vi "HFRR ADV v08 new software.vi"() -> ()   [LabVIEW 2025] (continued)
                n2706 = local read "String 37"() -> (w3531:string)
                n2707 = local read "String 36"() -> (w3528:string)
                n2708 = local read "String 38"() -> (w3525:string)
                n2709 = local read "String 39"() -> (w3522:string)
                n2710 = Match Pattern(string=w3552, regular expression=".dwm") -> (before substring=w3548:string)  [unwired: 1 in, 3 out]
                "before substring" <- w3548
                n2711 = local read "S 38"() -> (w3543:string)
                n2712 = local read "S 39"() -> (w3536:string)
                n2713 = local read "Temperature before test 2"() -> (w3572:dbl)
                n2714 = local read "Temperature after test 2"() -> (w3577:dbl)
                n2715 = local read "Humidity before test 2"() -> (w3558:dbl)
                n2716 = local read "Humidity after test 2"() -> (w3573:dbl)
                n2717 = local read "MWSD 2"() -> (w3569:dbl)
                n2718 = local read "WS1.4 2"() -> (w3585:dbl)
                n2719 = local read "HCF 2"() -> (w3581:dbl)
                n2720 = local read "AVP 2"() -> (w3570:dbl)
                n2721 = Concatenate Strings("1," ("string"), w3543) -> (w3542:string)
                n2722 = Concatenate Strings("2," ("string"), w3540) -> (w3539:string)
                n2723 = Concatenate Strings("3," ("string"), w3536) -> (w3538:string)
                n2724 = Concatenate Strings("4," ("string"), w3535) -> (w3534:string)
                n2725 = Concatenate Strings("5," ("string"), w3531) -> (w3532:string)
                n2726 = Concatenate Strings("6," ("string"), w3528) -> (w3529:string)
                n2727 = Concatenate Strings("7," ("string"), w3525) -> (w3526:string)
                n2728 = Concatenate Strings("8," ("string"), w3522) -> (w3523:string)
                n2729 = local read "Sample ID"() -> (w3590:string)
                n2730 = case shown="\"xlx\"" "Select File Type" {
                  tunnel: w3548 -> [w3593 w3595 w3597]
                  tunnel: [w3591 w3596 w3598] -> w3547
                  frame "xlx" {
                    n2731 = Concatenate Strings(w3593, ".xls" ("string")) -> (w3591:string)
                  }
                  frame "csv" {
                    n2732 = Concatenate Strings(w3595, ".csv" ("string")) -> (w3596:string)
                  }
                  frame "txt" {
                    n2733 = Concatenate Strings(w3597, ".txt" ("string")) -> (w3598:string)
                  }
                }
                n2734 = local read "Test Date"() -> (w3589:string)
                n2735 = local read "String 45"() -> (w3503:string)
                n2736 = local read "String 31"() -> (w3588:string)
                n2737 = local read "String 32"() -> (w3587:string)
                n2738 = local read "TITTLE"() -> (w3511:string)
                n2739 = Number To Fractional String(number=w3558, width (-)=i16 6, precision (6)=i16 2) -> (F-format string=w3557:string)  [unwired: 1 in]
                n2740 = Number To Fractional String(number=w3572, width (-)=i16 6, precision (6)=i16 2) -> (F-format string=w3578:string)  [unwired: 1 in]
                n2741 = Number To Fractional String(number=w3573, width (-)=i16 6, precision (6)=i16 2) -> (F-format string=w3571:string)  [unwired: 1 in]
                n2742 = Number To Fractional String(number=w3577, width (-)=i16 6, precision (6)=i16 2) -> (F-format string=w3576:string)  [unwired: 1 in]
                n2743 = Number To Fractional String(number=w3569, width (-)=i16 6, precision (6)=i16 2) -> (F-format string=w3567:string)  [unwired: 1 in]
                n2744 = Number To Fractional String(number=w3570, width (-)=i16 6, precision (6)=i16 2) -> (F-format string=w3568:string)  [unwired: 1 in]
                n2745 = Number To Fractional String(number=w3581, width (-)=i16 6, precision (6)=i16 2) -> (F-format string=w3582:string)  [unwired: 1 in]
                n2746 = Number To Fractional String(number=w3585, precision (6)=i16 2) -> (F-format string=w3586:string)  [unwired: 2 in]
                n2747 = local read "s.NO"() -> (w3505:string)
                n2748 = Concatenate Strings("=" ("string"), w3511) -> (w3510:string)
                n2749 = Concatenate Strings("S.No," ("string"), "                                       Parameters" ("string")) -> (w3516:string)
                n2750 = Concatenate Strings(w3583, w3542, w3557, w3583, w3539, w3578, w3583, w3538, w3571, w3583, w3534, w3576, w3583, w3532, w3567, w3583, w3529, w3568, w3583, w3526, w3582, w3583, w3523, w3586) -> (w3545:string)
                n2751 = Concatenate Strings(w3515, "," ("string"), w3503, w3505, w3504, w3587, w3590, w3504, w3588, w3589, w3515) -> (w3513:string)
                n2752 = local read "Tested by"() -> (w3519:string)
                n2753 = local read "String 33"() -> (w3520:string)
                n2754 = Concatenate Strings("," ("string"), "                                                                             " ("string")) -> (w3508:string)
                n2755 = Concatenate Strings(w3510, w3506, w3513, w3506, w3516, w3545, w3506, w3508, w3520, w3519) -> (→"export":string)
                n2756 = String To Path(string=w3547) -> (path=w3554:path)
                n2757 = local read "export"() -> (w3549:string)
                n2758 = call <vilib>:"Write Characters To File.vi"("append to file? (new file:F)"=FALSE, "character string"=w3549, "file path (dialog if empty)"=w3554) -> ()  [unwired: 2 in, 1 out]
              }
            }
          }
          frame Enabled {
          }
        }
        n2759 = case shown="True" "OK Button 17" {
          frame False {
          }
          frame True {
            (unwired) 0  # existing file
            w3807 = "Choose a datalog file to open"  # prompt
            n2760 = local write "OK Button 17"(FALSE ("OK Button 17")) -> ()
            n2761 = local read "String"() -> (w3802:string)
            n2762 = String To Path(string=w3802) -> (path=w3803:path)
            n2763 = File Dialog(6:"*.duf" ("pattern"), 7:w3807, 11:w3803) -> (0:w3794:errorcluster, 3:w3813:path)  [unwired: 4 in, 2 out]
            n2764 = Unbundle(w3794) -> ()  [unwired: 3 out]
            n2765 = Open/Create/Replace File "Open File"(file path (use dialog)=w3813) -> (refnum out=w3805:refnum<file>)  [unwired: 5 in, 2 out]
            n2766 = Strip Path(path=w3813) -> (name=w3811:string)  [unwired: 1 out]
            n2767 = Path To String(path=w3813) -> (string=w3796:string)
            n2768 = while {
              tunnel: w3805 -> [w3817]
              i -> [w3814]
              stop <- w3815 continue-if-true
              (unwired) TRUE ("line mode (F)")
              n2769 = Read from Text File "Read File"(file (use dialog)=w3817) -> (text=w3816:string)  [unwired: 3 in, 3 out]
              n2770 = local write "Numeric 16"(w3814) -> ()
              n2771 = String Length(string=w3816) -> (length=w3819:i32)
              n2772 = Greater?(x=w3819, y=1) -> (0:w3815:bool)
            }
            n2773 = local write "String 29"(w3796) -> ()
            n2774 = Search and Replace String(input string=w3796, search string=".duf", replace string=".dgf" ("replace string (\"\")")) -> (result string=→"String Indicator 4":string)  [unwired: 5 in, 3 out]
            n2775 = Match Pattern(string=w3811, regular expression=".dwm") -> (before substring=w3795:string)  [unwired: 1 in, 3 out]
            "String Indicator" <- w3795
            n2776 = Match Pattern(string=w3796, regular expression=".dwm" ("substring (\"\")")) -> (before substring=w3797:string)  [unwired: 1 in, 3 out]
            "String Indicator 3" <- w3797
            n2777 = local write "TITTLE 2"(w3795) -> ()
            n2778 = String To Path(string=w3797) -> (path=w3804:path)
            "path" <- w3804
            n2779 = call <vilib>:"Read Characters From File.vi"("file path (dialog if empty)"=w3804, "start of read offset (chars.:0)"=60 ("start of read offset (chars.: 0)")) -> ("character string"=→"String Indicator 2":string)  [unwired: 4 in, 3 out]
          }
        }
        n2780 = call <vilib>:"Query Available Printers.vi"() -> ("system configured printers"=w3496:string[])  [unwired: 9 in, 2 out]
        "System Configured Printers 2" <- w3496
        n2781 = local read "OK Button 16"() -> (w3493:bool)
        n2782 = case shown="True" "OK Button 16" {
          frame False {
          }
          frame True {
            n2783 = stacked-sequence {
              frame #0 {
                n2784 = local read "Numeric 16"() -> (w3821:i32)
                n2785 = local write "Numeric 10"(w3821) -> ()
              }
              frame #1 {
                n2786 = local read "S.NO"() -> (→"s.NO":string)
                n2787 = local read "String 29"() -> (w3825:string)
                n2788 = String To Path(string=w3825) -> (path=w3824:path)
                n2789 = Open/Create/Replace File "Open File"(file path (use dialog)=w3824) -> (refnum out=w3826:refnum<file>)  [unwired: 5 in, 2 out]
                n2790 = for {
                  N: 16 -> [_]
                  tunnel: w3826 -> [w3833]
                  i -> [w3829]
                  (unwired) TRUE ("line mode (F)")
                  n2791 = Read from Text File "Read File"(file (use dialog)=w3833) -> (text=w3827:string)  [unwired: 3 in, 3 out]
                  n2792 = Match Pattern(string=w3827, regular expression="(") -> (after substring=w3832:string)  [unwired: 1 in, 3 out]
                  n2793 = Match Pattern(string=w3832, regular expression=")") -> (before substring=w3828:string)  [unwired: 1 in, 3 out]
                  n2794 = case shown="1" w3829 {
                    tunnel: w3828 -> [w3834 w3835 _ _ w3836 w3837 w3838 w3840 w3842 w3844 w3846 w3848 w3850 w3852 _]
                    tunnel: w3827 -> [_ _ _ _ _ _ _ _ _ _ _ _ _ _ _]
                    frame 0 {
                      "TITTLE" <- w3834
                    }
                    frame 1 {
                      "Sample ID" <- w3835
                    }
                    frame 2 {
                    }
                    frame 3 {
                    }
                    frame 4 {
                      "Test Date" <- w3836
                    }
                    frame 5 {
                      "Tested by" <- w3837
                    }
                    frame 6 {
                      n2795 = Fract/Exp String To Number(string=w3838) -> (number=→"Humidity before test 2":dbl)  [unwired: 3 in, 1 out]
                    }
                    frame 7 {
                      n2796 = Fract/Exp String To Number(string=w3840) -> (number=→"Temperature before test 2":dbl)  [unwired: 3 in, 1 out]
                    }
                    frame 8 {
                      n2797 = Fract/Exp String To Number(string=w3842) -> (number=→"Humidity after test 2":dbl)  [unwired: 3 in, 1 out]
                    }
                    frame 9 {
                      n2798 = Fract/Exp String To Number(string=w3844) -> (number=→"Temperature after test 2":dbl)  [unwired: 3 in, 1 out]
                    }
                    frame 10 {
                      n2799 = Fract/Exp String To Number(string=w3846) -> (number=→"MWSD 2":dbl)  [unwired: 3 in, 1 out]
                    }
                    frame 11 {
                      n2800 = Fract/Exp String To Number(string=w3848) -> (number=→"AVP 2":dbl)  [unwired: 3 in, 1 out]
                    }
                    frame 12 {
                      n2801 = Fract/Exp String To Number(string=w3850) -> (number=→"HCF 2":dbl)  [unwired: 3 in, 1 out]
                    }
                    frame 13 {
                      n2802 = Fract/Exp String To Number(string=w3852) -> (number=→"WS1.4 2":dbl)  [unwired: 3 in, 1 out]
                    }
                    frame 14, Default {
                    }
                  }
                }
              }
              frame #2 {
              }
            }
            n2803 = local write "OK Button 16"(FALSE ("OK Button 13")) -> ()
          }
        }
        n2804 = Index Array(array=w3496, index="Select Printer 3") -> (element=w3498:string)
        "Selected Printer" <- w3498
        n2805 = case shown="True" w3493 {
          frame False {
          }
          frame True {
            n2806 = flat-sequence {
              frame #0 {
              }
              frame #1 {
                n2807 = Wait (ms)(milliseconds to wait=u32 100) -> ()  [unwired: 1 out]
              }
              frame #2 {
                n2808 = local write "OK Button 16"(FALSE ("Print 3")) -> ()
              }
            }
          }
        }
        n2809 = case shown="True" "Print" {
          tunnel: w3498 -> [_ w3790]
          frame False {
          }
          frame True {
            (unwired) i16 6 ("width (-)")
            (unwired) "TESTED BY : "
            (unwired) "TESTED DATE :"
            (unwired) "SAMPLE ID : "
            (unwired) "SAMPLE DESIGN : "
            w3748 = "\r"
            w3765 = "\r"
            # "add image"
            n2810 = local read "Sample ID"() -> (w3738:string)
            n2811 = local read "Tested by"() -> (w3741:string)
            n2812 = local read "String 34"() -> (w3728:string)
            n2813 = local read "String 45"() -> (w3708:string)
            n2814 = local read "String 35"() -> (w3723:string)
            n2815 = local read "String 37"() -> (w3721:string)
            n2816 = local read "String 32"() -> (w3743:string)
            n2817 = local read "String 36"() -> (w3718:string)
            n2818 = local read "String 31"() -> (w3742:string)
            n2819 = local read "Test Date"() -> (w3739:string)
            n2820 = local read "String 33"() -> (w3744:string)
            n2821 = local read "String 38"() -> (w3714:string)
            n2822 = local read "String 39"() -> (w3711:string)
            n2823 = local write "Print"(FALSE ("Print FF")) -> ()
            n2824 = local read "S 39"() -> (w3726:string)
            n2825 = local read "S 38"() -> (w3733:string)
            n2826 = local read "Temperature before test 2"() -> (w3764:dbl)
            n2827 = local read "Temperature after test 2"() -> (w3754:dbl)
            n2828 = local read "Humidity before test 2"() -> (w3779:dbl)
            n2829 = local read "Humidity after test 2"() -> (w3763:dbl)
            n2830 = local read "MWSD 2"() -> (w3768:dbl)
            n2831 = local read "WS1.4 2"() -> (w3746:dbl)
            n2832 = Concatenate Strings("2)" ("string"), w3728) -> (w3729:string)
            n2833 = Concatenate Strings("3)" ("string"), w3726) -> (w3727:string)
            n2834 = Concatenate Strings("1)" ("string"), w3733) -> (w3732:string)
            n2835 = Concatenate Strings("4)" ("string"), w3723) -> (w3724:string)
            n2836 = Concatenate Strings("5)" ("string"), w3721) -> (w3720:string)
            n2837 = Concatenate Strings("6)" ("string"), w3718) -> (w3717:string)
            n2838 = Concatenate Strings("7)" ("string"), w3714) -> (w3715:string)
            n2839 = Concatenate Strings("8)" ("string"), w3711) -> (w3712:string)
            n2840 = local read "HCF 2"() -> (w3750:dbl)
            n2841 = local read "AVP 2"() -> (w3767:dbl)
            n2842 = local read "s.NO"() -> (w3709:string)
            n2843 = call <vilib>:"New Report.vi"("report type"=enum16{"Standard Report", "HTML"}."Standard Report") -> ("report out"=w3788:refnum<class "NI_report.lvclass">, "error out"=w3787:errorcluster)  [unwired: 13 in]
            n2844 = local read "TITTLE"() -> (w3740:string)
            n2845 = Concatenate Strings(w3765, w3708, w3709, w3765, w3743, w3738, w3765, w3742, w3739, w3765, w3744, w3741, w3765) -> (w3758:string)
            "test by" <- w3758
            n2846 = Number To Fractional String(number=w3764, width (-)=i16 6, precision (6)=i16 2) -> (F-format string=w3753:string)  [unwired: 1 in]
            n2847 = Number To Fractional String(number=w3763, width (-)=i16 6, precision (6)=i16 2) -> (F-format string=w3766:string)  [unwired: 1 in]
            n2848 = Number To Fractional String(number=w3779, width (-)=i16 6, precision (6)=i16 2) -> (F-format string=w3784:string)  [unwired: 1 in]
            n2849 = Number To Fractional String(number=w3768, width (-)=i16 6, precision (6)=i16 2) -> (F-format string=w3770:string)  [unwired: 1 in]
            n2850 = Number To Fractional String(number=w3754, width (-)=i16 6, precision (6)=i16 2) -> (F-format string=w3755:string)  [unwired: 1 in]
            n2851 = Number To Fractional String(number=w3767, width (-)=i16 6, precision (6)=i16 2) -> (F-format string=w3769:string)  [unwired: 1 in]
            n2852 = Number To Fractional String(number=w3750, width (-)=i16 6, precision (6)=i16 2) -> (F-format string=w3749:string)  [unwired: 1 in]
            n2853 = Number To Fractional String(number=w3746, precision (6)=i16 2) -> (F-format string=w3745:string)  [unwired: 2 in]
            n2854 = call-dynamic "Set Report Header Text.vi"("report in"=w3788, "center header text"=w3740, "error in (no error)"=w3787) -> ("report out"=w3759:refnum<class "NI_report.lvclass">, "error out"=w3760:errorcluster)  [unwired: 11 in]
            n2855 = Concatenate Strings(w3748, w3732, w3784, w3748, w3729, w3753, w3748, w3727, w3766, w3748, w3724, w3755, w3748, w3720, w3770, w3748, w3717, w3769, w3748, w3715, w3749, w3748, w3712, w3745) -> (w3736:string)
            "export 2" <- w3736
            n2856 = call-poly <vilib>:"Append Report Text.vi"("report in"=w3759, "text"=w3758, "error in (no error)"=w3760) -> ("report out"=w3762:refnum<class "NI_report.lvclass">, "error out"=w3761:errorcluster)  [unwired: 9 in, 2 out]
            n2857 = local read "test by"() -> (w3735:string)
            n2858 = local read "TITTLE"() -> (w3737:string)
            n2859 = call-poly <vilib>:"Append Report Text.vi"("report in"=w3762, "error in (no error)"=w3761) -> ("report out"=w3783:refnum<class "NI_report.lvclass">, "error out"=w3781:errorcluster)  [unwired: 10 in, 2 out]
            n2860 = Concatenate Strings(w3737, w3736, w3735) -> (→"output":string)
            n2861 = call-poly <vilib>:"Append Report Text.vi"("report in"=w3783, "text"=w3736, "error in (no error)"=w3781) -> ("report out"=w3782:refnum<class "NI_report.lvclass">, "error out"=w3780:errorcluster)  [unwired: 9 in, 2 out]
            n2862 = call-dynamic "Print Report.vi"("report in"=w3782, "printer name (default)"=w3790, "error in (no error)"=w3780) -> ("report out"=w3792:refnum<class "NI_report.lvclass">, "error out"=w3793:errorcluster)  [unwired: 11 in]
            n2863 = call-dynamic "Dispose Report.vi"("report in"=w3792, "error in (no error)"=w3793) -> ()  [unwired: 13 in, 1 out]
          }
        }
        n2864 = case shown="True" "Print 2" {
          frame False {
          }
          frame True {
            n2865 = flat-sequence {
              frame #0 {
                n2866 = local read "s.NO"() -> (→"s.NO 2":string)
                n2867 = Wait (ms)(milliseconds to wait=u32 20) -> ()  [unwired: 1 out]
                n2868 = local read "Sample ID  3"() -> (→"Sample ID  6":string)
                n2869 = local read "Sample ID  4"() -> (→"Sample ID  7":string)
                n2870 = local read "Sample ID"() -> (→"Sample ID  2":string)
                n2871 = local read "Tested by"() -> (→"Tested by 2":string)
                n2872 = local read "Test Date"() -> (→"Test Date 2":string)
                n2873 = local read "Humidity after test 3"() -> (→"Humidity after test 4":dbl)
                n2874 = local read "Ref A Test Date :"() -> (→"TITTLE 4":string)
                n2875 = local read "Temperature before test 3"() -> (w3615:dbl)
                n2876 = local read "Temperature before test 3"() -> (→"Temperature after test 5":dbl)
                n2877 = local read "Temperature after test 3"() -> (→"Temperature after test 4":dbl)
                n2878 = local read "Humidity before test 3"() -> (→"Humidity before test 4":dbl)
                n2879 = local write "Temperature before test 3"(w3615) -> ()
                n2880 = local read "image data"() -> (w3606:T14)
                n2881 = String To Path(string="C:\\LAB-IQ\\im\\Temp_resized.jpg") -> (path=w3607:path)
                "path 2" <- w3607
                n2882 = call <vilib>:"Write JPEG File.vi"("image data"=w3606, "path to JPEG file"=w3607) -> ()  [unwired: 8 in, 2 out]
                "Ref A Test Date :" <- "Ref A Test Date :"
                "Ref B Test Date :" <- "Ref B Test Date :"
                "Ref B Scar Value :" <- "Ref B Scar Value :"
                "Ref A Scar Value :" <- "Ref A Scar Value :"
              }
              frame #1 {
                (unwired) HTML_Report_Image_Alignment."MIDDLE" ("alignment (default)")
                w3643 = u16 0 items=["portrait", "landscape"] ("orientation (portrait)")
                (unwired) HTML_Report_Image_Alignment."ABSMIDDLE" ("alignment (default)")
                (unwired) "TESTED BY : "
                (unwired) "TESTED DATE :"
                (unwired) "SAMPLE ID : "
                (unwired) "SAMPLE DESIGN : "
                w3676 = "\r"
                # "add image"
                n2883 = Wait (ms)(milliseconds to wait=u32 20) -> ()  [unwired: 1 out]
                n2884 = local read "Sample ID  2"() -> (w3669:string)
                n2885 = local read "Wear Scar X"() -> (w3641:dbl)
                "Length ( microns ) 2" <- w3641
                n2886 = local read "Wear Scar Y"() -> (w3640:dbl)
                "Wear Scar Y ( microns ) :" <- w3640
                n2887 = local read "Test Date 2"() -> (w3670:string)
                n2888 = local read "Tested by 2"() -> (w3671:string)
                n2889 = local read "String 46"() -> (w3667:string)
                n2890 = local read "String 48"() -> (w3673:string)
                n2891 = local read "String 47"() -> (w3672:string)
                n2892 = local read "String 49"() -> (w3674:string)
                n2893 = local read "String 10"() -> (w3627:string)
                n2894 = local read "s.NO 2"() -> (w3668:string)
                n2895 = Add(x=w3641, y=w3640) -> (x+y=w3639:dbl)
                n2896 = call <vilib>:"New Report.vi"("report type"=enum16{"Standard Report", "HTML"}."HTML") -> ("report out"=w3647:refnum<class "NI_report.lvclass">, "error out"=w3645:errorcluster)  [unwired: 13 in]
                n2897 = Concatenate Strings(w3676, w3667, w3668, w3676, w3673, w3669, w3676, w3672, w3670, w3676, w3674, w3671, w3676) -> (→"test by 2":string)
                n2898 = Concatenate Strings("C:\\LAB-IQ\\Data\\" ("string"), w3627, ".jpg" ("string")) -> ()  [unwired: 1 out]
                n2899 = Divide(x=w3639, y=2.0) -> (x/y=→"Mean Wear ( microns) :":dbl)
                n2900 = call-dynamic "Set Report Orientation.vi"("report in"=w3647, "orientation (portrait)"=w3643, "error in (no error)"=w3645) -> ("report out"=w3646:refnum<class "NI_report.lvclass">, "error out"=w3644:errorcluster)  [unwired: 11 in]
                n2901 = for {
                  N: 5 -> [_]
                  tunnel: w3646 -> [w3697]
                  tunnel: [w3696] -> w3625
                  tunnel: w3644 -> [w3695]
                  tunnel: [w3694] -> w3624
                  n2902 = call-dynamic "Set Report Tab Width.vi"("report in"=w3697, "error in (no error)"=w3695) -> ("report out"=w3696:refnum<class "NI_report.lvclass">, "error out"=w3694:errorcluster)  [unwired: 12 in]
                }
                n2903 = local read "TITTLE"() -> (w3642:string)
                n2904 = call-dynamic "Set Report Header Text.vi"("report in"=w3625, "center header text"=w3642, "error in (no error)"=w3624) -> ("report out"=w3663:refnum<class "NI_report.lvclass">, "error out"=w3662:errorcluster)  [unwired: 11 in]
                n2905 = for {
                  N: 1 -> [_]
                  tunnel: [w3701] -> w3649
                  tunnel: [w3700] -> w3648
                  tunnel: w3663 -> [w3699]
                  tunnel: w3662 -> [w3698]
                  n2906 = call-dynamic "New Report Line.vi"("report in"=w3699, "error in (no error)"=w3698) -> ("report out"=w3701:refnum<class "NI_report.lvclass">, "error out"=w3700:errorcluster)  [unwired: 12 in]
                }
                n2907 = for {
                  N: 2 -> [_]
                  tunnel: [w3693] -> w3655
                  tunnel: [w3692] -> w3654
                  tunnel: w3649 -> [w3691]
                  tunnel: w3648 -> [w3690]
                  n2908 = call-dynamic "New Report Line.vi"("report in"=w3691, "error in (no error)"=w3690) -> ("report out"=w3693:refnum<class "NI_report.lvclass">, "error out"=w3692:errorcluster)  [unwired: 12 in]
                }
                n2909 = for {
                  N: 25 -> [_]
                  tunnel: w3655 -> [w3689]
                  tunnel: w3654 -> [w3687]
                  tunnel: [w3688] -> w3658
                  tunnel: [w3686] -> w3657
                  n2910 = call-dynamic "Set Report Tab Width.vi"("report in"=w3689, "error in (no error)"=w3687) -> ("report out"=w3688:refnum<class "NI_report.lvclass">, "error out"=w3686:errorcluster)  [unwired: 12 in]
                }
                n2911 = control-ref of="Tab Control 9"() -> (w3653:refnum<vi>)
                n2912 = call-dynamic "Append Control Image to Report.vi"("report in"=w3658, "alignment (default)"=HTML_Report_Image_Alignment."ABSMIDDLE", "ctrl reference"=w3653, "error in (no error)"=w3657) -> ("report out"=w3652:refnum<class "NI_report.lvclass">, "error out"=w3651:errorcluster)  [unwired: 8 in, 2 out]
                n2913 = for {
                  N: 3 -> [_]
                  tunnel: [w3685] -> w3636
                  tunnel: [w3684] -> w3635
                  tunnel: w3652 -> [w3683]
                  tunnel: w3651 -> [w3682]
                  n2914 = call-dynamic "New Report Line.vi"("report in"=w3683, "error in (no error)"=w3682) -> ("report out"=w3685:refnum<class "NI_report.lvclass">, "error out"=w3684:errorcluster)  [unwired: 12 in]
                }
                n2915 = for {
                  N: 100 -> [_]
                  tunnel: w3636 -> [w3681]
                  tunnel: w3635 -> [w3679]
                  tunnel: [w3680] -> w3632
                  tunnel: [w3678] -> w3630
                  n2916 = call-dynamic "Set Report Tab Width.vi"("report in"=w3681, "error in (no error)"=w3679) -> ("report out"=w3680:refnum<class "NI_report.lvclass">, "error out"=w3678:errorcluster)  [unwired: 12 in]
                }
                n2917 = String To Path(string="C:\\LAB-IQ\\im\\Temp_resized.jpg") -> (path=w3622:path)
                n2918 = call-poly <vilib>:"Append Image to Report.vi"("report in"=w3632, "path or URL of image"=w3622, "error in (no error)"=w3630) -> ("report out"=w3631:refnum<class "NI_report.lvclass">, "error out"=w3629:errorcluster)  [unwired: 9 in, 2 out]
                n2919 = call-poly <vilib>:"Open HTML Report in Browser.vi"("report in"=w3631, "error in (no error)"=w3629) -> ("report out"=w3666:refnum<class "NI_report.lvclass">, "error out"=w3665:errorcluster)  [unwired: 11 in, 1 out]
                n2920 = call-dynamic "Dispose Report.vi"("report in"=w3666, "error in (no error)"=w3665) -> ()  [unwired: 13 in, 1 out]
              }
              frame #2 {
              }
              frame #3 {
                n2921 = disable-structure shown="Disabled" {
                  frame Disabled {
                    n2922 = local read "String 10"() -> (w3706:string)
                    n2923 = Concatenate Strings("C:\\LAB-IQ-NXT\\Data\\" ("string"), w3706, ".jpg" ("string")) -> (w3704:string)
                    n2924 = String To Path(string=w3704) -> (path=w3703:path)
                    n2925 = Delete(path (use dialog)=w3703) -> ()  [unwired: 4 in, 3 out]
                  }
                  frame Enabled {
                  }
                }
                n2926 = local write "Print 2"(FALSE ("Print")) -> ()
              }
            }
          }
        }
      }
    }
    n2927 = property on="SetTemp" class="DigNum (strict)"("Disabled"=w1649) -> ()  [unwired: 2 in, 2 out]
    n2928 = Multiply(x=w1639, y=w1641) -> (x*y=w1640:dbl)
    n2929 = local read "MWSD"() -> (w1638:dbl)
    n2930 = Add(x=w1640, y=w1638) -> (x+y=→"WS1.4":dbl)
    n2931 = Wait (ms)(milliseconds to wait=u32 50) -> ()  [unwired: 1 out]
    n2932 = Wait (ms)(milliseconds to wait=u32 50) -> ()  [unwired: 1 out]
    n2933 = local read "Quit"() -> (w1637:bool)
  }
  n2934 = VISA Close(VISA resource name=w52, error in (no error)=w51) -> (error out=w49:errorcluster)
  n2935 = call <vilib>:"Clear Errors.vi"("error in (no error)"=w49) -> ()  [unwired: 5 in, 2 out]
  n2936 = VISA Close(VISA resource name=w37, error in (no error)=w36) -> ()  [unwired: 1 out]
  n2937 = while {
    tunnel: [w3865] -> w46
    shift-right: [w3858] -> _
    shift-left: 0.0 -> [w3861]
    shift-right: [w3857] -> _
    shift-left: 0.0 -> [w3860]
    shift-right: [w3856] -> _
    shift-left: 400.0 ("vc_cmd") -> [w3859]
    stop <- w3865 stop-if-true
    # "PID LOGIC"
    n2938 = local read "RUN"() -> (w3863:bool)
    n2939 = local read "Auto Start Test"() -> (w3862:bool)
    n2940 = local read "START TEMP"() -> (w3854:bool)
    n2941 = Or(x=w3863, y=w3862) -> (x .or. y?=w3864:bool)
    n2942 = And(x=w3864, y=w3854) -> (x .and. y?=w3855:bool)
    n2943 = Wait (ms)(milliseconds to wait=u32 20) -> ()  [unwired: 1 out]
    n2944 = case shown="True" w3855 {
      tunnel: [400.0 ("out_vc_cmd") w3885] -> w3856
      tunnel: [w3868 w3887] -> w3857
      tunnel: [w3868 w3886] -> w3858
      tunnel: w3861 -> [_ w3876]
      tunnel: w3860 -> [_ w3875]
      tunnel: w3859 -> [_ w3874]
      frame False {
        w3868 = 0.0 ("error_out")
      }
      frame True {
        n2945 = local read "Set Strk"() -> (w3871:dbl)
        n2946 = local read "LVDT STROKE"() -> (w3869:dbl)
        n2947 = Add(x=w3871, y="Add up Stroke") -> (x+y=w3872:dbl)
        n2948 = formula code="// Zero-Hardcode Explicit Positional-Form PID Engine\n// Inputs: target_stroke, measured_stroke, dt, prev_error, integral_accumulator_in, prev_vc_cmd\n//         kp, ki, kd, max_step_change, max_amplitude, min_amplitude, startup_cmd\n// Outputs: vc_cmd, error_out, out_error, integral_accumulator_out, out_vc_cmd\n\n// 1. Calculate Tracking Error\nfloat current_error = target_stroke - measured_stroke;\nerror_out = current_error;\n\n// 2. Compute Proportional Term\nfloat p_term = kp * current_error;\n\n// 3. Compute Derivative Term\nfloat d_term = 0.0;\nif (dt > 0.0) {\n    d_term = kd * ((current_error - prev_error) / dt);\n}\n\n// 4. Update and Accumulate Integral Term\nfloat current_integral = integral_accumulator_in + (current_error * dt);\nfloat i_term = ki * current_integral;\n\n// 5. Calculate Ideal Target Command\nfloat ideal_command = startup_cmd + p_term + i_term + d_term;\n\n// 6. Anti-Windup Protection (Back-calculation method)\nif (ideal_command > max_amplitude) {\n    float excess = ideal_command - max_amplitude;\n    if (ki > 0.0) {\n        current_integral -= excess / ki;\n    }\n    ideal_command = max_amplitude;\n} else if (ideal_command < min_amplitude) {\n    float excess = ideal_command - min_amplitude;\n    if (ki > 0.0) {\n        current_integral -= excess / ki;\n    }\n    ideal_command = min_amplitude;\n}\n\n// 7. Apply Loop Rate Limiting (Protects voice coil from large voltage steps)\nfloat raw_adjustment = ideal_command - prev_vc_cmd;\n\nif (raw_adjustment > max_step_change) {\n    raw_adjustment = max_step_change;\n} else if (raw_adjustment < -max_step_change) {\n    raw_adjustment = -max_step_change;\n}\n\nfloat next_vc_cmd = prev_vc_cmd + raw_adjustment;\n\n// Final Output Safety Safeguard Clamping\nif (next_vc_cmd > max_amplitude) {\n    next_vc_cmd = max_amplitude;\n} else if (next_vc_cmd < min_amplitude) {\n    next_vc_cmd = min_amplitude;\n}\n\n// 8. Map to Shift Registers for memory persistence\nvc_cmd = next_vc_cmd;\nout_error = current_error;                     \nintegral_accumulator_out = current_integral;  \nout_vc_cmd = next_vc_cmd;"("target_stroke"=w3872, "measured_stroke"=w3869, "dt"="dt", "integral_accumulator_in"=w3875, "prev_error"=w3876, "prev_vc_cmd"=w3874, "kp"="kp", "ki"="ki", "kd"="kd", "max_step_change"="max_step_change", "max_amplitude"="max_amplitude", "min_amplitude"="min_amplitude", "startup_cmd"="startup_cmd") -> ("vc_cmd"=w3891:dbl, "out_error"=w3886:dbl, "integral_accumulator_out"=w3887:dbl, "out_vc_cmd"=w3885:dbl)  [unwired: 1 out]
        "output Vpp" <- w3891
        n2949 = Number To Fractional String(number=w3891, precision (6)=i16 1) -> (F-format string=w3889:string)  [unwired: 2 in]
        n2950 = Concatenate Strings("DAC;" ("string"), w3889) -> (w3873:string)
        n2951 = local write "Command"(w3873) -> ()
        "prev_error" <- w3876
        "integral_accumulator_in" <- w3875
        "prev_vc_cmd" <- w3874
      }
    }
    n2952 = local read "Quit"() -> (w3865:bool)
  }
  n2953 = Or(x=w42, y=w41) -> (x .or. y?=w43:bool)
  n2954 = Or(x=w39, y=w43) -> (x .or. y?=w48:bool)
  n2955 = control-ref of="new picture"() -> ()  [unwired: 1 out]
  n2956 = Or(x=w54, y=w48) -> (x .or. y?=w45:bool)
  n2957 = Or(x=w45, y=w46) -> (x .or. y?=w40:bool)
  n2958 = while {
    tunnel: [w3892] -> w53
    i -> [w3899]
    stop <- w3892 stop-if-true
    n2959 = local read "Quit"() -> (w3892:bool)
    n2960 = Equal To 0?(x=w3899) -> (x = 0?=w3897:bool)
    n2961 = call "Elapsed Time3"("Time Target (s)"=45.0, "Auto Reset"=TRUE) -> ("Time has Elapsed"=w3896:bool)  [unwired: 10 in, 7 out]
    n2962 = Wait (ms)(milliseconds to wait=u32 50) -> ()  [unwired: 1 out]
    n2963 = Or(x=w3896, y=w3897) -> (x .or. y?=w3898:bool)
    n2964 = case shown="True" w3898 {
      frame False {
      }
      frame True {
        n2965 = call <vilib>:"System Exec.vi"("run minimized? (F)"=TRUE, "error in (no error)"="error in (no error)", "command line"="powercfg.exe -change -monitor-timeout-ac 0") -> ("error out"=w3910:errorcluster)  [unwired: 5 in, 3 out]
        n2966 = call <vilib>:"System Exec.vi"("run minimized? (F)"=TRUE, "error in (no error)"=w3910, "command line"="powercfg.exe -change -disk-timeout-ac 0") -> ("error out"=w3909:errorcluster)  [unwired: 5 in, 3 out]
        n2967 = call <vilib>:"System Exec.vi"("run minimized? (F)"=TRUE, "error in (no error)"=w3909, "command line"="powercfg.exe -change -standby-timeout-ac 0") -> ("error out"=w3908:errorcluster)  [unwired: 5 in, 3 out]
        n2968 = call <vilib>:"System Exec.vi"("run minimized? (F)"=TRUE, "error in (no error)"=w3908, "command line"="powercfg.exe -change -hibernate-timeout-ac 0") -> ("error out"=w3907:errorcluster)  [unwired: 5 in, 3 out]
        n2969 = call <vilib>:"Simple Error Handler.vi"("error in (no error)"=w3907) -> ("error out"=w3913:errorcluster)  [unwired: 4 in, 4 out]
        n2970 = call <vilib>:"Clear Errors.vi"("error in (no error)"=w3913) -> ("error out"=→"error out":errorcluster)  [unwired: 5 in, 1 out]
      }
    }
  }
  n2971 = Compound Arithmetic op=OR(w56, w40, w53) -> (w55:bool)
  n2972 = flat-sequence {
    tunnel: w55 -> [_]
    tunnel: [w3915] -> w18
    tunnel: w18 -> [_]
    frame #0 {
      n2973 = call "CLOSE CONNECTION.vi"() -> ("error out"=w3915:errorcluster)  [unwired: 11 in]
    }
    frame #1 {
      n2974 = Quit LabVIEW(quit? (T)=TRUE) -> ()
      n2975 = local write "Quit"(FALSE ("EXIT")) -> ()
    }
  }
  n2976 = property on="Heater Button" class="Bool (strict)"("Visible"=TRUE) -> ()  [unwired: 2 in, 2 out]
  n2977 = disable-structure shown="Disabled" {
    disable-tunnel: _ -> [w3921 _]
    disable-tunnel: _ -> [w3918 _]
    disable-tunnel: _ -> [w3919 _]
    frame Disabled {
      n2978 = disable-structure shown="Disabled" {
        disable-tunnel: [w3928 _] -> w3920
        frame Disabled {
          n2979 = while {
            shift-right: [w3970] -> w3926
            shift-left: errorcluster {"status"=TRUE, "code"=0, "source"="Init"} ("error out") -> [w3935]
            shift-right: [w3969] -> w3925
            shift-left: _ -> [w3936]
            shift-right: [w3968] -> _
            shift-left: "" -> [w3967]
            tunnel: [w3929] -> w3928
            shift-right: ["Set Rh"] -> _
            shift-left: 0.0 ("Set Rh") -> [w3961]
            tunnel: [w3938] -> _
            i -> [w3938]
            stop <- w3929 stop-if-true
            n2980 = flat-sequence {
              tunnel: w3935 -> [w3973]
              tunnel: [w3973] -> w3934
              frame #0 {
                n2981 = Wait (ms)(milliseconds to wait=u32 200) -> ()  [unwired: 1 out]
              }
            }
            n2982 = local read "Com Port 3"() -> (w3937:refnum<visa-resource-name>)
            n2983 = local read "Humidity Str Rec"() -> (w3939:string)
            n2984 = Not Equal?(x="Set Rh", y=w3961) -> (x != y?=w3966:bool)
            n2985 = Number To Decimal String(number="Set Rh") -> (decimal integer string=w3964:string)  [unwired: 1 in]
            n2986 = Not Equal?(x=w3937, y=w3936) -> (x != y?=w3932:bool)
            n2987 = Concatenate Strings("#setPoint00" ("string"), w3964) -> (w3965:string)
            n2988 = case shown="False" w3966 {
              tunnel: w3965 -> [_ w3985]
              frame False {
                n2989 = local read "Humidity"() -> (w3982:bool)
                n2990 = case shown="True" w3982 {
                  frame False {
                    n2991 = local write "Humidity Str Send"("stop" ("Humidity Str Send")) -> ()
                  }
                  frame True {
                    n2992 = local write "Humidity Str Send"("start" ("Humidity Str Send")) -> ()
                  }
                }
              }
              frame True {
                n2993 = local write "Humidity Str Send"(w3985) -> ()
              }
            }
            n2994 = Or(x=w3932) -> (y=w3930:bool, x .or. y?=w3931:bool)
            n2995 = String Subset(string=w3939, offset (0)=7) -> (substring=w3954:string)  [unwired: 1 in]
            n2996 = Match Pattern(string=w3939, regular expression="?") -> (offset past match=w3957:i32)  [unwired: 1 in, 3 out]
            n2997 = Match Pattern(string=w3939, regular expression="v") -> (offset past match=w3960:i32)  [unwired: 1 in, 3 out]
            n2998 = case shown="True" w3931 {
              tunnel: w3934 -> [w3971 _]
              tunnel: [w3971 errorcluster {"status"=TRUE, "code"=0, "source"="Init"} ("error out")] -> w3933
              frame False {
              }
              frame True {
              }
            }
            n2999 = Equal?(x=w3957, y=-1) -> (x = y?=w3941:bool)
            n3000 = Match Pattern(string=w3954, regular expression="g") -> (after substring=w3955:string, offset past match=w3946:i32)  [unwired: 1 in, 2 out]
            n3001 = Match Pattern(string=w3954, regular expression="y") -> (after substring=w3953:string, offset past match=w3947:i32)  [unwired: 1 in, 2 out]
            n3002 = Greater?(x=w3947, y=w3946) -> (0:w3952:bool)
            n3003 = Greater Or Equal To 0?(x=w3947) -> (x >= 0?=w3944:bool)
            n3004 = Greater Or Equal To 0?(x=w3946) -> (x >= 0?=w3945:bool)
            n3005 = Or(x=w3944, y=w3945) -> (x .or. y?=w3943:bool)
            n3006 = Greater Or Equal To 0?(x=w3960) -> (x >= 0?=w3942:bool)
            n3007 = Select(t=w3953, s=w3952, f=w3955) -> (s? t:f=w3948:string)
            n3008 = case shown="Error" w3933 {
              selector: w3933 -> [w3998 w4044]
              tunnel: [w3996 w4037] -> w3970
              tunnel: w3936 -> [w3999 w4043]
              tunnel: [w3997 w4046] -> w3969
              tunnel: w3967 -> [w3986 w4045]
              tunnel: [w3993 w4045] -> w3968
              frame No Error {
                n3009 = call "Elapsed Time7"() -> ("Time has Elapsed"=w3992:bool)  [unwired: 12 in, 7 out]
                n3010 = Not Equal?(x="Humidity Str Send", y=w3986) -> (x != y?=w3988:bool)
                n3011 = Or(x=w3988, y=w3992) -> (x .or. y?=w3991:bool)
                n3012 = Select(t="Humidity Str Send", s=w3988, f="vals" ("regular expression")) -> (s? t:f=w3987:string)
                n3013 = Or(x=w3991, y="Send") -> (x .or. y?=w3995:bool)
                n3014 = case shown="True" w3995 {
                  tunnel: [w4002 w4007] -> w3996
                  tunnel: w3999 -> [w4001 w4015]
                  tunnel: w3998 -> [w4002 w4014]
                  tunnel: [w4001 w4008] -> w3997
                  tunnel: w3987 -> [_ w4013]
                  tunnel: [w4000 w4004] -> w3993
                  tunnel: "Humidity Str Send" -> [_ w4005]
                  tunnel: w3988 -> [_ w4006]
                  tunnel: w3986 -> [w4000 w4003]
                  frame False {
                  }
                  frame True {
                    n3015 = flat-sequence {
                      tunnel: w4015 -> [w4023]
                      tunnel: w4014 -> [w4022]
                      tunnel: w4013 -> [w4019]
                      tunnel: [w4021] -> w4012
                      tunnel: [w4020] -> w4011
                      tunnel: w4012 -> [w4026]
                      tunnel: w4011 -> [w4025]
                      tunnel: [w4026] -> w4010
                      tunnel: [w4025] -> w4009
                      tunnel: w4010 -> [w4033]
                      tunnel: w4009 -> [w4032]
                      tunnel: [w4031] -> w4008
                      tunnel: [w4030] -> w4007
                      frame #0 {
                        n3016 = local write "Ser Led"(TRUE ("Boolean 4")) -> ()
                        n3017 = Concatenate Strings(w4019, "\r") -> (w4018:string)
                        n3018 = VISA Write(VISA resource name=w4023, write buffer=w4018, error in (no error)=w4022) -> (VISA resource name out=w4021:refnum<visa-resource-name>, error out=w4020:errorcluster)  [unwired: 1 out]
                      }
                      frame #1 {
                        n3019 = Wait (ms)(milliseconds to wait="wait") -> ()  [unwired: 1 out]
                      }
                      frame #2 {
                        w4028 = FALSE ("Send")
                        n3020 = property class="Instr"(reference=w4033, error in=w4032) -> (reference out=w4034:refnum<visa-resource-name>, error out=w4035:errorcluster, "Serial Settings:Number of Bytes at Serial Port"=w4027:u32)
                        n3021 = local write "Send"(w4028) -> ()
                        n3022 = local write "Ser Led"(w4028) -> ()
                        n3023 = VISA Read(VISA resource name=w4034, byte count=w4027, error in (no error)=w4035) -> (VISA resource name out=w4031:refnum<visa-resource-name>, read buffer=→"Humidity Str Rec":string, error out=w4030:errorcluster)  [unwired: 1 out]
                      }
                    }
                    n3024 = Select(t=w4005, s=w4006, f=w4003) -> (s? t:f=w4004:string)
                  }
                }
              }
              frame Error {
                w4051 = u16 0 items=["None"=0, "XON/XOFF"=1, "RTS/CTS"=2, "DTR/DSR"=4] ("flow control")
                w4047 = u16 0 items=["None", "Odd", "Even", "Mark", "Space"] ("parity")
                w4050 = u16 10 items=["1.0"=10, "1.5"=15, "2.0"=20] ("stop bits")
                n3025 = VISA Close(VISA resource name=w4043, error in (no error)=w4044) -> (error out=w4042:errorcluster)
                n3026 = local write "humid"("" ("humid")) -> ()
                n3027 = local write "Humidity Str Rec"("" ("Humidity Str Rec")) -> ()
                n3028 = call <vilib>:"Clear Errors.vi"("error in (no error)"=w4042) -> ("error out"=w4041:errorcluster)  [unwired: 5 in, 1 out]
                n3029 = local read "Com Port 3"() -> (w4040:refnum<visa-resource-name>)
                n3030 = call-poly "VISA Configure Serial Port"("VISA resource name"=w4040, "timeout (10sec)"=u32 1000, "termination char\n(0xA = '\\n' = LF)"=u8 10 ("termination char\n(0xA = '\\n' = LF)"), "Enable Termination\nChar (T)"=FALSE ("Enable Termination Char (T)"), "data bits (8)"=u16 8 ("data bits"), "parity (0:none)"=w4047, "error in (no error)"=w4041, "stop bits (10: 1 bit)"=w4050, "flow control (0:none)"=w4051) -> ("VISA resource name out"=w4046:refnum<visa-resource-name>, "baud rate (9600)"=w4038:u32, "error out"=w4037:errorcluster)  [unwired: 4 in]
              }
            }
            n3031 = Compound Arithmetic op=AND(w3942, w3941, w3943) -> (w3940:bool)
            n3032 = case shown="True" w3940 {
              tunnel: w3939 -> [_ _]
              tunnel: w3948 -> [_ w3978]
              frame False {
              }
              frame True {
                w3976 = " " ("regular expression")
                n3033 = Match Pattern(string=w3978, regular expression=" ") -> (after substring=w3980:string)  [unwired: 1 in, 3 out]
                n3034 = Match Pattern(string=w3980, regular expression=w3976) -> (before substring=→"humid":string, after substring=w3977:string)  [unwired: 1 in, 2 out]
                n3035 = Match Pattern(string=w3977, regular expression=w3976) -> (before substring=→"temp_@Rh sensor":string)  [unwired: 1 in, 3 out]
              }
            }
            n3036 = local read "Quit"() -> (w3929:bool)
          }
          n3037 = VISA Close(VISA resource name=w3925, error in (no error)=w3926) -> (error out=w3922:errorcluster)
          n3038 = call <vilib>:"Clear Errors.vi"("error in (no error)"=w3922) -> ()  [unwired: 5 in, 2 out]
        }
        frame Enabled {
        }
      }
    }
    frame Enabled {
    }
  }
  n3039 = while {
    tunnel: [w4058] -> _
    i -> [w4058]
    stop <- w4054 stop-if-true
    # "Langauage selection"
    n3040 = Equal?(x="Lan flag", y=22.0) -> ()  [unwired: 1 out]
    n3041 = disable-structure shown="Disabled" {
      frame Disabled {
        n3042 = stacked-sequence {
          frame #0 {
            n3043 = case shown="\"Russian\"" "Language Selection" {
              tunnel: [0 1] -> w4060
              frame "English", Default {
              }
              frame "Russian" {
              }
            }
            n3044 = for {
              N: 130 -> [_]
              tunnel: "Table" -> [w4069]
              tunnel: w4060 -> [w4068]
              i -> [w4067]
              n3045 = Index Array(array=w4069, index (row)=w4067, index (col)=w4068) -> (element=w4066:string)
              n3046 = case shown="123" w4067 {
                tunnel: w4066 -> [w4070 w4071 _ w4072 w4073 w4074 w4075 w4076 w4077 w4078 w4079 w4080 w4081 w4082 w4083 w4084 w4085 w4086 w4087 w4088 w4089 w4090 w4091 w4092 w4093 w4094 w4095 w4096 w4097 _ _ w4098 w4099 w4100 w4101 w4102 w4103 w4112 w4119 w4126 w4133 w4137 w4140 w4143 w4145 w4147 w4148 w4149 w4150 w4151 w4152 w4153 w4154 w4155 w4156 w4157 w4158 w4159 w4160 w4161 w4162 w4163 w4164 w4165 w4166 w4167 w4168 w4169 w4170 w4171 w4172 w4173 w4174 w4175 w4176 w4177 w4178 w4179 w4180 w4181 w4182 w4183 w4184 w4185 w4186 w4187 w4188 w4189 w4190 w4191 w4192 w4193 w4194 w4195 w4196 w4197 w4198 w4199 w4200 w4201 w4202 w4203 w4204 w4205 w4206 _ w4207 w4208 w4209 w4210 w4211 w4212 w4213 w4214 w4215 w4216 w4217 w4218 w4219 _ w4220 w4221 w4222 w4223 w4224 w4225 _]
                frame 0 {
                  n3047 = local write "S"(w4070) -> ()
                }
                frame 1 {
                  n3048 = local write "S 2"(w4071) -> ()
                }
                frame 2 {
                }
                frame 3 {
                  n3049 = local write "S 4"(w4072) -> ()
                }
                frame 4 {
                  n3050 = property on="FILE" class="Str"("Caption.Text"=w4073) -> ()  [unwired: 2 in, 2 out]
                }
                frame 5 {
                  n3051 = property on="Fuel Discription :" class="Str"("Caption.Text"=w4074) -> ()  [unwired: 2 in, 2 out]
                }
                frame 6 {
                  n3052 = property on="Remarks :" class="Str"("Caption.Text"=w4075) -> ()  [unwired: 2 in, 2 out]
                }
                frame 7 {
                  n3053 = property on="Save & Continue" class="Bool (strict)"("Boolean Text.Text"=w4076) -> ()  [unwired: 2 in, 2 out]
                }
                frame 8 {
                }
                frame 9 {
                  n3054 = property on="Set Hz" class="DigNum (strict)"("Caption.Text"=w4078) -> ()  [unwired: 2 in, 2 out]
                }
                frame 10 {
                  "String 3" <- w4079
                }
                frame 11 {
                  n3055 = property on="NORMAL LOAD" class="DigNum (strict)"("Caption.Text"=w4080) -> ()  [unwired: 2 in, 2 out]
                }
                frame 12 {
                  "String 5" <- w4081
                }
                frame 13 {
                  n3056 = property on="Set Temp" class="DigNum (strict)"("Caption.Text"=w4082) -> ()  [unwired: 2 in, 2 out]
                }
                frame 14 {
                  n3057 = local write "S 15"(w4083) -> ()
                }
                frame 15 {
                  n3058 = property on="Set Rh" class="DigNum (strict)"("Caption.Text"=w4084) -> ()  [unwired: 2 in, 2 out]
                }
                frame 16 {
                  "String 13" <- w4085
                  "String 26" <- w4085
                }
                frame 17 {
                  n3059 = local write "S 18"(w4086) -> ()
                }
                frame 18 {
                  "String 17" <- w4087
                }
                frame 19 {
                  n3060 = property on="test time" class="DigNum (strict)"("Caption.Text"=w4088) -> ()  [unwired: 2 in, 2 out]
                }
                frame 20 {
                  "String 18" <- w4089
                  "String 22" <- w4089
                }
                frame 21 {
                  n3061 = property on="Elapsed time" class="DigNum (strict)"("Caption.Text"=w4090) -> ()  [unwired: 2 in, 2 out]
                }
                frame 22 {
                  n3062 = property on="Samplingtime 2" class="DigNum (strict)"("Caption.Text"=w4091) -> ()  [unwired: 2 in, 2 out]
                }
                frame 23 {
                  "String 21" <- w4092
                }
                frame 24 {
                  n3063 = property on="Countdown" class="DigNum (strict)"("Caption.Text"=w4093) -> ()  [unwired: 2 in, 2 out]
                }
                frame 25 {
                  n3064 = property on="Countdown 2" class="DigNum (strict)"("Caption.Text"=w4094) -> ()  [unwired: 2 in, 2 out]
                }
                frame 26 {
                  n3065 = property on="Engage" class="Bool (strict)"("Boolean Text.Text"=w4095) -> ()  [unwired: 2 in, 2 out]
                }
                frame 27 {
                  n3066 = property on="Boolean  4" class="Bool (strict)"("Boolean Text.Text"=w4096) -> ()  [unwired: 2 in, 2 out]
                }
                frame 28 {
                  n3067 = property on="Test \nStatus" class="Bool (strict)"("Boolean Text.Text"=w4097) -> ()  [unwired: 2 in, 2 out]
                }
                frame 29 {
                }
                frame 30 {
                }
                frame 31 {
                }
                frame 32 {
                  n3068 = property on="RSTCOF" class="Bool"("Boolean Text.Text"=w4099) -> ()  [unwired: 2 in, 2 out]
                  n3069 = property on="RST FF" class="Bool"("Boolean Text.Text"=w4099) -> ()  [unwired: 2 in, 2 out]
                  n3070 = property on="RST TEMP" class="Bool"("Boolean Text.Text"=w4099) -> ()  [unwired: 2 in, 2 out]
                  n3071 = property on="RSTV1 3" class="Bool"("Boolean Text.Text"=w4099) -> ()  [unwired: 2 in, 2 out]
                  n3072 = property on="rstv2" class="Bool"("Boolean Text.Text"=w4099) -> ()  [unwired: 2 in, 2 out]
                  n3073 = property on="RSTV1 2" class="Bool"("Boolean Text.Text"=w4099) -> ()  [unwired: 2 in, 2 out]
                  n3074 = property on="RST CP" class="Bool"("Boolean Text.Text"=w4099) -> ()  [unwired: 2 in, 2 out]
                }
                frame 33 {
                  "S 61" <- w4100
                }
                frame 34 {
                  "String 23" <- w4101
                }
                frame 35 {
                  n3075 = property on="Rh Before" class="DigNum (strict)"("Caption.Text"=w4102) -> ()  [unwired: 2 in, 2 out]
                }
                frame 36 {
                  n3076 = Match Pattern(string=w4103, regular expression=",") -> (before substring=→"bs":string, after substring=→"as":string)  [unwired: 1 in, 2 out]
                  n3077 = property on="Rh After" class="DigNum (strict)"("Caption.Text"=w4103) -> ()  [unwired: 2 in, 2 out]
                }
                frame 37 {
                  n3078 = Match Pattern(string=w4112, regular expression=",") -> (before substring=w4111:string, after substring=w4110:string)  [unwired: 1 in, 2 out]
                  "bs" <- w4111
                  "as" <- w4110
                  n3079 = Concatenate Strings(w4111, w4110) -> (w4107:string)
                  n3080 = property on="Humidity before test 2" class="DigNum (strict)"("Caption.Text"=w4107) -> ()  [unwired: 2 in, 2 out]
                  n3081 = property on="Humidity before test" class="DigNum (strict)"("Caption.Text"=w4107) -> ()  [unwired: 2 in, 2 out]
                  n3082 = Concatenate Strings(w4107, "=" ("string")) -> (w4108:string)
                  n3083 = local write "S 38"(w4108) -> ()
                }
                frame 38 {
                  n3084 = Match Pattern(string=w4119, regular expression=",") -> (before substring=w4118:string, after substring=w4117:string)  [unwired: 1 in, 2 out]
                  "bs" <- w4118
                  "as" <- w4117
                  n3085 = Concatenate Strings(w4118, w4117) -> (w4114:string)
                  n3086 = property on="Humidity after test 2" class="DigNum (strict)"("Caption.Text"=w4114) -> ()  [unwired: 2 in, 2 out]
                  n3087 = Concatenate Strings(w4114, "=" ("string")) -> (w4116:string)
                  n3088 = property on="Humidity after test" class="DigNum (strict)"("Caption.Text"=w4114) -> ()  [unwired: 2 in, 2 out]
                  n3089 = local write "S 39"(w4116) -> ()
                }
                frame 39 {
                  n3090 = Match Pattern(string=w4126, regular expression=",") -> (before substring=w4125:string, after substring=w4124:string)  [unwired: 1 in, 2 out]
                  "bs" <- w4125
                  "as" <- w4124
                  n3091 = Concatenate Strings(w4125, w4124) -> (w4121:string)
                  n3092 = property on="Temperature before test 2" class="DigNum (strict)"("Caption.Text"=w4121) -> ()  [unwired: 2 in, 2 out]
                  n3093 = property on="Temperature before test" class="DigNum (strict)"("Caption.Text"=w4121) -> ()  [unwired: 2 in, 2 out]
                  n3094 = Concatenate Strings(w4121, "=" ("string")) -> (→"String 34":string)
                }
                frame 40 {
                  n3095 = Match Pattern(string=w4133, regular expression=",") -> (before substring=w4132:string, after substring=w4131:string)  [unwired: 1 in, 2 out]
                  "bs" <- w4132
                  "as" <- w4131
                  n3096 = Concatenate Strings(w4132, w4131) -> (w4128:string)
                  n3097 = property on="Temperature after test 2" class="DigNum (strict)"("Caption.Text"=w4128) -> ()  [unwired: 2 in, 2 out]
                  n3098 = Concatenate Strings(w4128, "=" ("string")) -> (→"String 35":string)
                  n3099 = property on="Temperature after test" class="DigNum (strict)"("Caption.Text"=w4128) -> ()  [unwired: 2 in, 2 out]
                }
                frame 41 {
                  n3100 = property on="AVP" class="DigNum (strict)"("Caption.Text"=w4137) -> ()  [unwired: 2 in, 2 out]
                  n3101 = property on="AVP 2" class="DigNum (strict)"("Caption.Text"=w4137) -> ()  [unwired: 2 in, 2 out]
                  n3102 = Concatenate Strings(w4137, "=" ("string")) -> (→"String 36":string)
                }
                frame 42 {
                  n3103 = property on="MWSD" class="DigNum (strict)"("Caption.Text"=w4140) -> ()  [unwired: 2 in, 2 out]
                  n3104 = property on="MWSD 2" class="DigNum (strict)"("Caption.Text"=w4140) -> ()  [unwired: 2 in, 2 out]
